vi "CS-4 Error Status.vi"(2 "error in (no error)":errorcluster, 3 "VI name":string, 4 "VISA session":refnum<visa-resource-name>) -> (0 "error out":errorcluster, 1 "dup VISA session":refnum<visa-resource-name>)   [LabVIEW 2016]
doc: "CS-4 Error Status.vi reads the Status Byte and checks for events in the Event Status Register. The Event Status Enable register must previously be set as demonstrated in CS-4 Operate.vi.\n\nIf enabled events are indicated, an error is set in the error cluster and reported to the calling application. The following error codes are defined:\n\n -1301: \"CS-4 Execution Error\" occurs when a command recognized by the CS-4 command parser can not be executed. This may be the result of a controlling command while in menu or local mode or a bad command parameter. \n -1302: \"CS-4 Command Error\" occurs if an invalid command or a command with an invalid parameter is received by the CS-4.\n -1303: \"Undefined Error\" is not presently used.\n -1304: \"CS-4 Query Error\" is generated under the conditions specified in IEEE Std 488.2-1992.\n -1305: \"CS-4 in Menu or Local\" is not decoded by this VI, but is included here for completeness. See CS-4 Status.vi for the generation of this error."
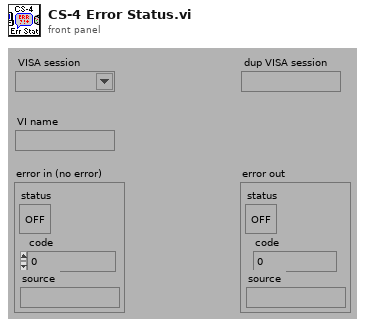
[diagram p1: front panel]
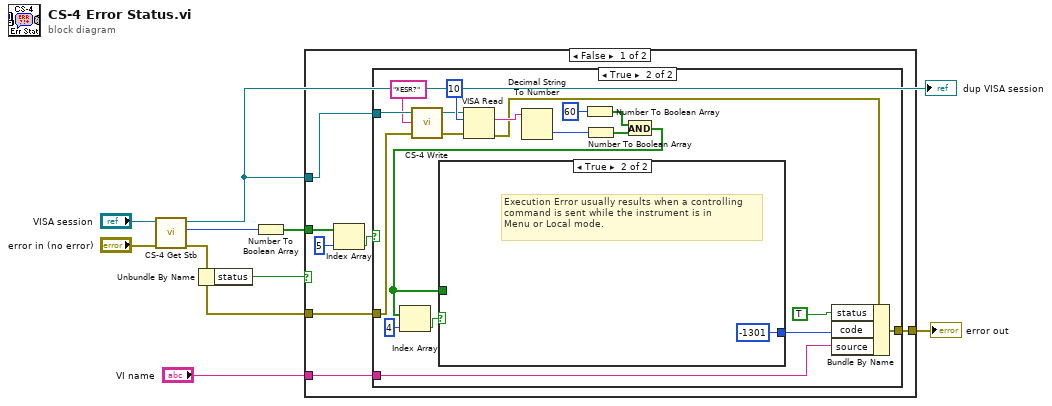
[diagram p0: block diagram]
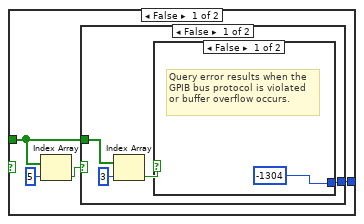
[diagram p3: hidden frame]
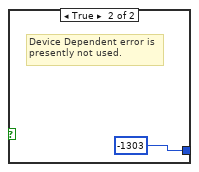
[diagram p4: hidden frame]
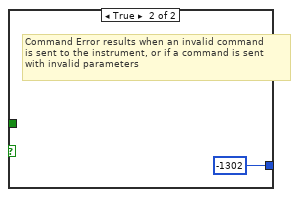
[diagram p5: hidden frame]
diagram:
  n1 = call "CS-4 Get Stb.vi"("error in (no error)"="error in (no error)", "VISA session"="VISA session") -> ("error out"=w2:errorcluster, "stb"=w1:i32, "dup VISA session"=w3:refnum<visa-resource-name>)  [unwired: 2 in, 1 out]
  "dup VISA session" <- w3
  n2 = Unbundle By Name(w2) -> ("status"=w6:bool)
  n3 = Number To Boolean Array(number=w1) -> (Boolean array=w9:bool[])
  n4 = case shown="False" w6 {
    tunnel: w2 -> [w13 w49]
    tunnel: [w12 w49] -> w8
    tunnel: w9 -> [w16 _]
    tunnel: w3 -> [w11 _]
    tunnel: "VI name" -> [w10 _]
    frame False {
      n5 = Index Array(array=w16, index=5) -> (element=w14:bool)
      n6 = case shown="True" w14 {
        tunnel: w13 -> [w17 w35]
        tunnel: [w17 w23] -> w12
        tunnel: w11 -> [_ w36]
        tunnel: w10 -> [_ w20]
        frame False {
        }
        frame True {
          n7 = call "CS-4 Write.vi"("error in (no error)"=w35, "write buffer (\"\")"="*ESR?" ("write buffer (\"\")"), "VISA session"=w36) -> ("error out"=w31:errorcluster, "dup VISA session"=w32:refnum<visa-resource-name>)  [unwired: 1 out]
          n8 = VISA Read(VISA resource name=w32, byte count=u32 10 ("byte count (0)"), error in (no error)=w31) -> (read buffer=w30:string, error out=w22:errorcluster)  [unwired: 2 out]
          n9 = Decimal String To Number(string=w30) -> (number=w27:i32)  [unwired: 2 in, 1 out]
          n10 = Number To Boolean Array(number=60) -> (Boolean array=w24:bool[])
          n11 = Number To Boolean Array(number=w27) -> (Boolean array=w26:bool[])
          n12 = And(x=w24, y=w26) -> (x .and. y?=w18:bool[])
          n13 = Index Array(array=w18, index=4) -> (element=w25:bool)
          n14 = case shown="True" w25 {
            tunnel: [w37 -1301] -> w19
            tunnel: w18 -> [w38 _]
            frame False {
              n15 = Index Array(array=w38, index=5) -> (element=w39:bool)
              n16 = case shown="False" w39 {
                tunnel: w38 -> [w43 _]
                tunnel: [w41 -1302] -> w37
                frame False {
                  n17 = Index Array(array=w43, index=3) -> (element=w42:bool)
                  n18 = case shown="False" w42 {
                    tunnel: [-1304 -1303] -> w41
                    frame False {
                      # "Query error results when the\nGPIB bus protocol is violated\nor buffer overflow occurs."
                    }
                    frame True {
                      # "Device Dependent error is\npresently not used."
                    }
                  }
                }
                frame True {
                  # "Command Error results when an invalid command\nis sent to the instrument, or if a command is sent\nwith invalid parameters"
                }
              }
            }
            frame True {
              # "Execution Error usually results when a controlling\ncommand is sent while the instrument is in \nMenu or Local mode."
            }
          }
          n19 = Bundle By Name(cluster=w22, "status"=TRUE, "code"=w19, "source"=w20) -> (w23:errorcluster)
        }
      }
    }
    frame True {
    }
  }
  "error out" <- w8
